vi "Sequence Init.vi"(8 "error in (no error)":errorcluster, 11 "DriverMasterSync in":refnum<class "DriverMasterSync.lvclass">) -> (0 "error out":errorcluster, 3 "DriverMasterSync out":refnum<class "DriverMasterSync.lvclass">)   [LabVIEW 2014, in "DriverMasterSync.lvlib" / "DriverMasterSync.lvclass"]
uses:
  DriverMasterSync.lvclass
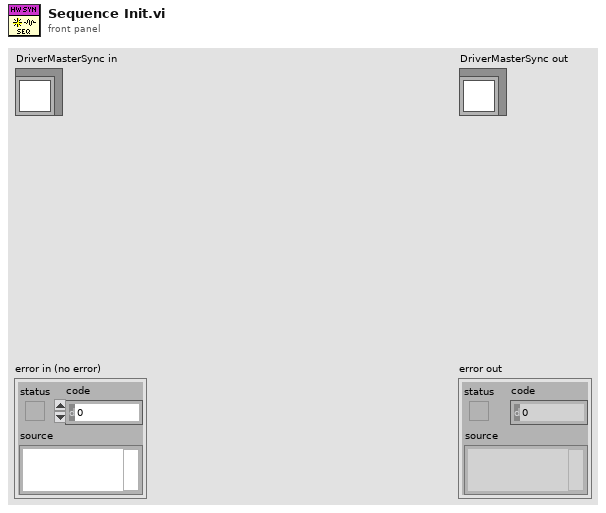
[diagram p1: front panel]
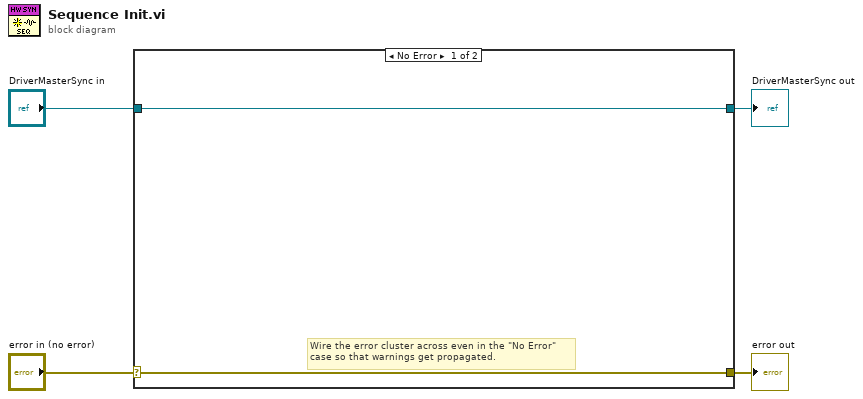
[diagram p0: block diagram]
diagram:
  n1 = case shown="No Error" "error in (no error)" {
    selector: "error in (no error)" -> [w5 w8]
    tunnel: [w5 w8] -> w3
    tunnel: [w6 w7] -> w1
    tunnel: "DriverMasterSync in" -> [w6 w7]
    frame No Error {
      # "Wire the error cluster across even in the \"No Error\"\ncase so that warnings get propagated."
    }
    frame Error {
    }
  }
  "error out" <- w3
  "DriverMasterSync out" <- w1
